vi "Log Data.vi"(7 "Command":T1, 8 "error in (no error)":errorcluster, 10 "Zone Setup Array":cluster{"Zone Selector":string, "Timing":dbl}[](array[cluster]), 11 "file path":path) -> (0 "error out":errorcluster, 2 "Array":cluster{"Zone Selector":string, "Timing":dbl}[](array[cluster]))   [LabVIEW 2013]
uses:
  Controls/Read Write States.ctl
  <vilib>/Utility/file.llb/Read From Spreadsheet File (string).vi
  <vilib>/Utility/file.llb/Write To Spreadsheet File (string).vi
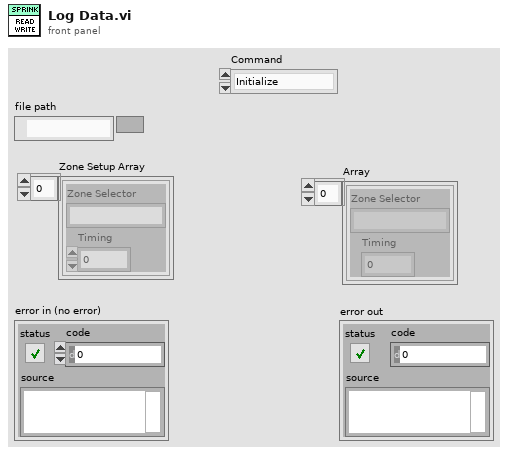
[diagram p1: front panel]
types:
  T1 = typedef "Read Write States.ctl" = enum16{"Initialize", "Read", "Write", "Stop"}
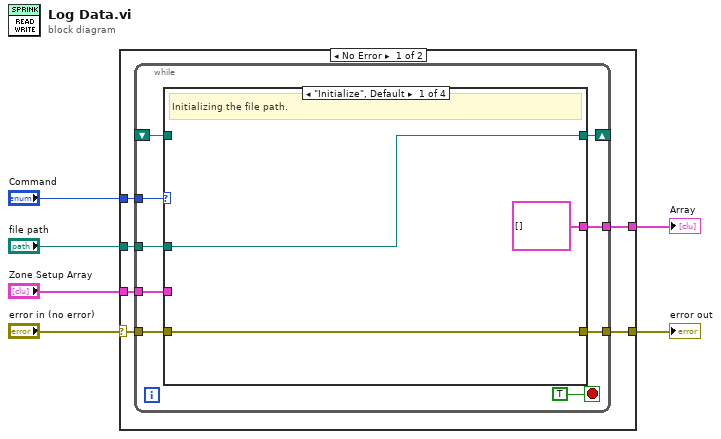
[diagram p0: block diagram]
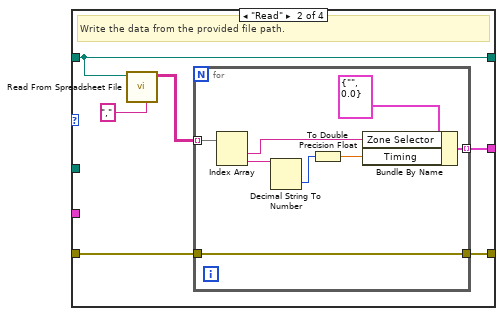
[diagram p2: hidden frame]
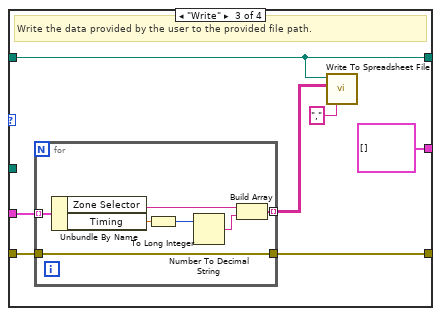
[diagram p3: hidden frame]
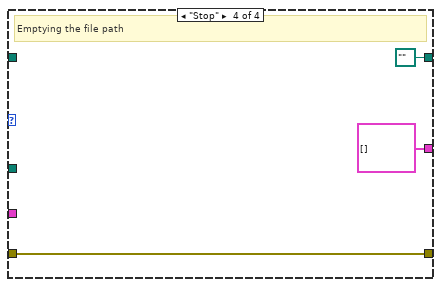
[diagram p4: hidden frame]
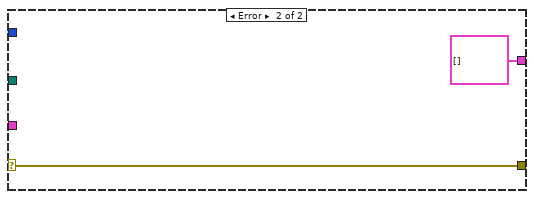
[diagram p5: hidden frame]
diagram:
  n1 = case shown="No Error" "error in (no error)" {
    selector: "error in (no error)" -> [w9 w57]
    tunnel: "Command" -> [w12 _]
    tunnel: "file path" -> [w11 _]
    tunnel: [w10 cluster{"Zone Selector":string, "Timing":dbl}[] []] -> w3
    tunnel: [w8 w57] -> w5
    tunnel: "Zone Setup Array" -> [w7 _]
    frame No Error {
      n2 = while {
        tunnel: w12 -> [w20]
        tunnel: w11 -> [w19]
        shift-right: [w18] -> _
        shift-left: _ -> [w17]
        tunnel: [w16] -> w10
        tunnel: w9 -> [w15]
        tunnel: [w14] -> w8
        tunnel: w7 -> [w13]
        stop <- TRUE stop-if-true
        n3 = case shown="\"Initialize\", Default" w20 {
          tunnel: w19 -> [w24 _ _ _]
          tunnel: [w24 w30 w45 path "" ("file path")] -> w18
          tunnel: w17 -> [_ w30 w45 _]
          tunnel: [cluster{"Zone Selector":string, "Timing":dbl}[] [] w29 cluster{"Zone Selector":string, "Timing":dbl}[] [] cluster{"Zone Selector":string, "Timing":dbl}[] []] -> w16
          tunnel: w15 -> [w23 w26 w41 w53]
          tunnel: [w23 w25 w42 w53] -> w14
          tunnel: w13 -> [_ _ w44 _]
          frame "Initialize", Default {
            # "Initializing the file path."
          }
          frame "Read" {
            # "Write the data from the provided file path."
            n4 = call-poly <vilib>:"Read From Spreadsheet File.vi"("delimiter (\\t)"="," ("delimiter (\\t)"), "file path (dialog if empty)"=w30) -> ("all rows"=w27:string[][])  [unwired: 5 in, 4 out]
            n5 = for {
              tunnel: [w38] -> w29 mode=indexing
              tunnel: w27 -> [w36] mode=indexing
              tunnel: w26 -> [w32]
              tunnel: [w32] -> w25
              n6 = Index Array(array=w36) -> (element #1=w35:string, element #2=w34:string)  [unwired: 2 in]
              n7 = Decimal String To Number(string=w34) -> (number=w31:i32)  [unwired: 2 in, 1 out]
              n8 = To Double Precision Float(number=w31) -> (double precision float=w33:dbl)
              n9 = Bundle By Name(cluster=cluster{"Zone Selector":string, "Timing":dbl} {"Zone Selector"="", "Timing"=0.0} ("Zone Selector"), "Zone Selector"=w35, "Timing"=w33) -> (w38:cluster{"Zone Selector":string, "Timing":dbl})
            }
          }
          frame "Write" {
            # "Write the data provided by the user to the provided file path."
            n10 = for {
              tunnel: w44 -> [w52] mode=indexing
              tunnel: [w47] -> w43 mode=indexing
              tunnel: [w46] -> w42
              tunnel: w41 -> [w46]
              n11 = Unbundle By Name(w52) -> ("Zone Selector"=w51:string, "Timing"=w49:dbl)
              n12 = To Long Integer(number=w49) -> (32bit integer=w48:i32)
              n13 = Number To Decimal String(number=w48) -> (decimal integer string=w50:string)  [unwired: 1 in]
              n14 = Build Array(w51, w50) -> (w47:string[])
            }
            n15 = call-poly <vilib>:"Write To Spreadsheet File.vi"("delimiter (\\t)"="," ("delimiter (\\t)"), "2D data"=w43, "file path (dialog if empty)"=w45) -> ()  [unwired: 5 in, 1 out]
          }
          frame "Stop" {
            # "Emptying the file path"
          }
        }
      }
    }
    frame Error {
    }
  }
  "error out" <- w5
  "Array" <- w3
